vi "Inventory Cluster to String Array.vi"(1 "Component Line":T1) -> (0 "Array":string[](array[string]))   [LabVIEW 2013]
uses:
  Controls/Add Component Line.ctl
  Controls/Components.ctl
  Controls/Component Sub Type.ctl
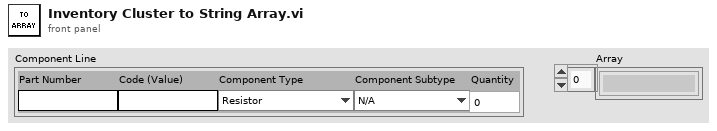
[diagram p1: front panel]
types:
  T1 = typedef "Add Component Line.ctl" = cluster{"Part Number":string, "Code (Value)":string, "Component Type":T2, "Component Subtype":T3, "Quantity":u32}
  T2 = typedef "Components.ctl" = enum16{"Resistor", "Capacitor", "Diode", "Voltage Regulator", "Transistors", "ICs"}
  T3 = typedef "Component Sub Type.ctl" = enum16{"N/A", "Carbon", "Variable - Trimmer", "Variable - Pot", "Ceramic", "Electrolitic", "Zenner", "TO-92", "TO-220", "NPN", "PNP", "CMOS", "Processor"}
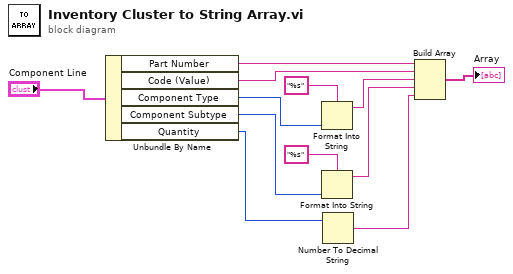
[diagram p0: block diagram]
diagram:
  n1 = Unbundle By Name("Component Line") -> ("Part Number"=w2:string, "Code (Value)"=w3:string, "Component Type"=w6:T2, "Component Subtype"=w7:T3, "Quantity"=w11:u32)
  n2 = Format Into String(format string="%s", w6) -> (resulting string=w4:string)  [unwired: 2 in, 1 out]
  n3 = Format Into String(format string="%s", w7) -> (resulting string=w5:string)  [unwired: 2 in, 1 out]
  n4 = Number To Decimal String(number=w11) -> (decimal integer string=w12:string)  [unwired: 1 in]
  n5 = Build Array(w2, w3, w4, w5, w12) -> (→"Array":string[])
